vi "Create All Message Queues.vi"(8 "error in":errorcluster) -> (0 "error out":errorcluster, 3 "Message Queues out":T1)   [LabVIEW 2022 SP3, in "Message Queue.lvlib"]
doc: "This VI creates and initializes all the message queues for your application. If your application requires more than one message queue, right-click the \"Message Queues\" constant above and select Open Type Def. Add the new Message Queue(s) to the type definition, then initialize them in this VI."
uses:
  Message Queue.lvlib
  All Message Queues.ctl
  Message Cluster.ctl
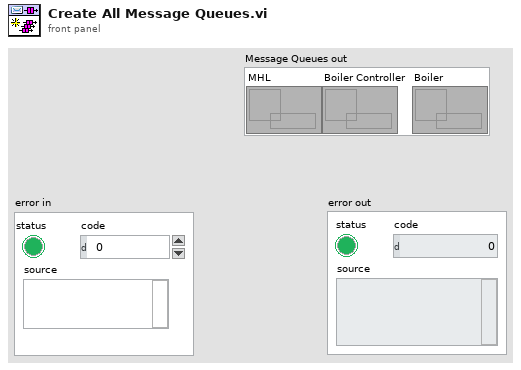
[diagram p1: front panel]
types:
  T1 = typedef "Message Queue.lvlib/All Message Queues.ctl" = cluster{"MHL":refnum<queue>, "Boiler Controller":refnum<queue>, "Boiler":refnum<queue>}
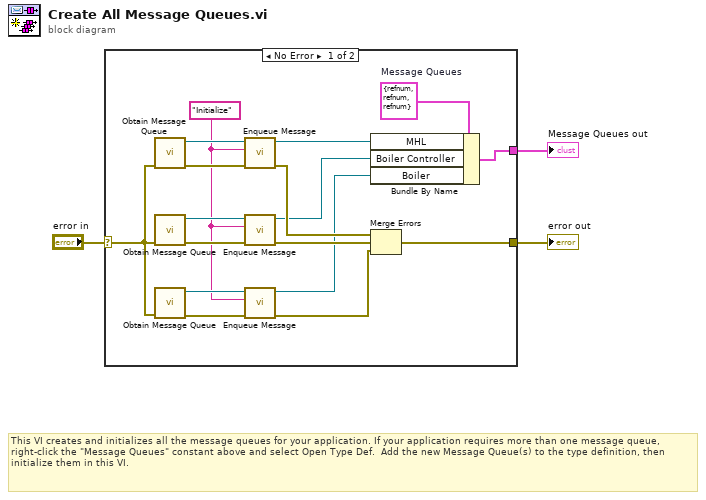
[diagram p0: block diagram]
diagram:
  # "This VI creates and initializes all the message queues for your application. If your application requires more than one message queue, right-click the \"Message Queues\" constant above and select Open Type Def.  Add the new Message Queue(s) to the type definition, then initialize them in this VI."
  n1 = case shown="No Error" "error in" {
    selector: "error in" -> [w10 w21]
    tunnel: [w13 w21] -> w2
    tunnel: [w19 _] -> w1
    frame No Error {
      w7 = "Initialize" ("Message")
      w20 = T1 {"MHL"=refnum, "Boiler Controller"=refnum, "Boiler"=refnum}  # Message Queues
      n2 = call "Obtain Message Queue.vi"("error in"=w10) -> ("error out"=w16:errorcluster, "Message Queue"=w17:refnum<queue>)  [unwired: 9 in]
      n3 = call "Obtain Message Queue.vi"("error in"=w10) -> ("error out"=w18:errorcluster, "Message Queue"=w14:refnum<queue>)  [unwired: 9 in]
      n4 = call "Obtain Message Queue.vi"("error in"=w10) -> ("error out"=w9:errorcluster, "Message Queue"=w8:refnum<queue>)  [unwired: 9 in]
      n5 = call "Enqueue Message.vi"("error in"=w16, "Message"=w7, "Message Queue"=w17) -> ("error out"=w11:errorcluster, "dup Message Queue"=w15:refnum<queue>)  [unwired: 7 in]
      n6 = call "Enqueue Message.vi"("error in"=w18, "Message"=w7, "Message Queue"=w14) -> ("error out"=w12:errorcluster, "dup Message Queue"=w4:refnum<queue>)  [unwired: 7 in]
      n7 = call "Enqueue Message.vi"("error in"=w9, "Message"=w7, "Message Queue"=w8) -> ("error out"=w5:errorcluster, "dup Message Queue"=w6:refnum<queue>)  [unwired: 7 in]
      n8 = Bundle By Name(cluster=w20, "MHL"=w15, "Boiler Controller"=w4, "Boiler"=w6) -> (w19:T1)
      n9 = Merge Errors(w11, w12, w5) -> (w13:errorcluster)
    }
    frame Error {
    }
  }
  "error out" <- w2
  "Message Queues out" <- w1
